vi "Import_Param.vi"() -> (0 "Calparam":sgl[](array[numeric]), 1 "Zero Offset":sgl, 2 "Fullscale":sgl, 3 "Initial Tare":sgl[](array[numeric]))   [LabVIEW 2018]
uses:
  <vilib>/Utility/file.llb/Read Delimited Spreadsheet (DBL).vi
panel:
  out "Samples":i64
  out "STD":i64
  out "ERMS":i64
  out "Offset":i64
  out "Gain":i64
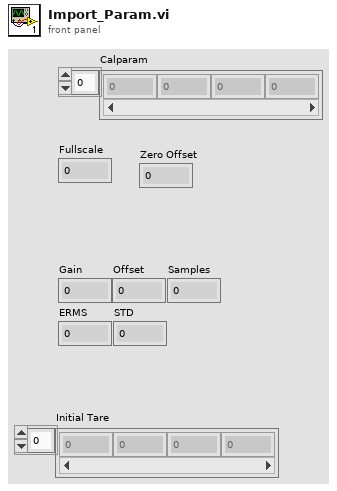
[diagram p1: front panel]
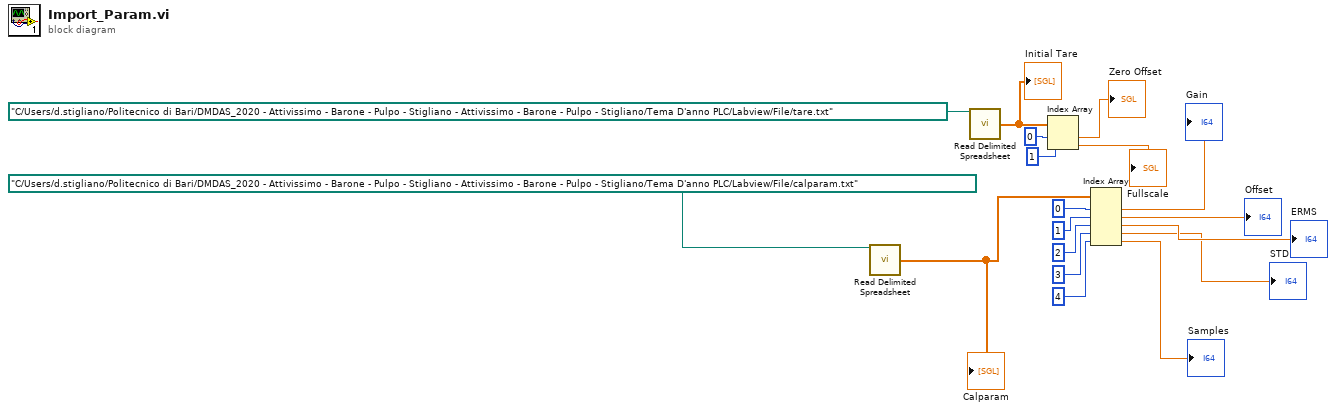
[diagram p0: block diagram]
diagram:
  n1 = call-poly <vilib>:"Read Delimited Spreadsheet.vi"("file path (dialog if empty)"=path "C:/Users/d.stigliano/Politecnico di Bari/DMDAS_2020 - Attivissimo - Barone - Pulpo - Stigliano - Attivissimo - Barone - Pulpo - Stigliano/Tema D'anno PLC/Labview/File/calparam.txt") -> ("first row"=w12:dbl[])  [unwired: 9 in, 5 out]
  "Calparam" <- w12
  n2 = call-poly <vilib>:"Read Delimited Spreadsheet.vi"("file path (dialog if empty)"=path "C:/Users/d.stigliano/Politecnico di Bari/DMDAS_2020 - Attivissimo - Barone - Pulpo - Stigliano - Attivissimo - Barone - Pulpo - Stigliano/Tema D'anno PLC/Labview/File/tare.txt") -> ("first row"=w16:dbl[])  [unwired: 9 in, 5 out]
  "Initial Tare" <- w16
  n3 = Index Array(array=w16, index #1=0 ("index"), index #2=1 ("index")) -> (element #1=→"Zero Offset":dbl, element #2=→"Fullscale":dbl)
  n4 = Index Array(array=w12, index #1=0 ("index"), index #2=1 ("index"), index #3=2 ("index"), index #4=3 ("index"), index #5=4 ("index")) -> (element #1=→"Gain":dbl, element #2=→"Offset":dbl, element #3=→"ERMS":dbl, element #4=→"STD":dbl, element #5=→"Samples":dbl)
